vi "Fire Delay Event.vi"(8 "error in (no error)":errorcluster, 10 "Delay mS":i32, 11 "MuxPanel in":refnum<class "MuxPanel.lvclass">) -> (0 "error out":errorcluster, 3 "MuxPanel out":refnum<class "MuxPanel.lvclass">)   [LabVIEW 2022 SP3, in "TouchControl.lvlib" / "MuxPanel.lvclass"]
uses:
  MuxPanel.lvclass
  MuxPanel.lvclass/MuxPanel.ctl
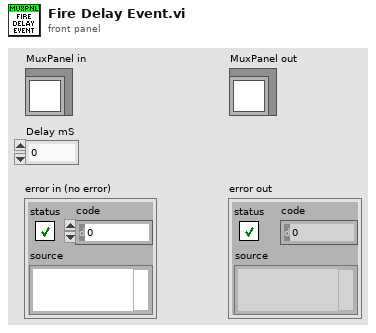
[diagram p1: front panel]
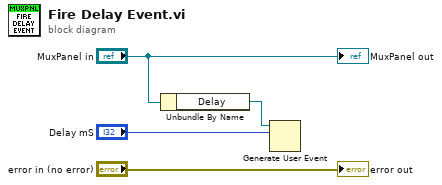
[diagram p0: block diagram]
diagram:
  n1 = Unbundle By Name("MuxPanel in") -> ("Delay"=w2:refnum<user-event>)
  n2 = Generate User Event(user event=w2, event data cluster="Delay mS") -> ()  [unwired: 2 in, 2 out]
  "error out" <- "error in (no error)"
  "MuxPanel out" <- "MuxPanel in"
